vi "Do Mutate.vi"(8 "error in":errorcluster, 10 "IGene in":refnum<class "IGene.lvclass">, 11 "Binary Mutator in":refnum<class "Binary Mutator.lvclass">) -> (0 "error out":errorcluster, 2 "IGene out":refnum<class "IGene.lvclass">, 3 "Binary Mutator out":refnum<class "Binary Mutator.lvclass">)   [LabVIEW 2016, in "Binary Mutator.lvclass"]
uses:
  Binary Mutator.lvclass
  C:/Users/J51654/My Projects/Evolutionary Programming/GA Framework/GA Core/GA Core.lvclass
  IGene/IGene.lvclass
  GA Core.lvclass/GA Core.ctl
  IGene/Children/Binary/Binary Gene.lvclass
  C:/Users/J51654/My Projects/Evolutionary Programming/GA Framework/IGene/IGene.lvclass
  IGene/Children/Binary/Binary Gene.lvclass/Binary Gene.ctl
  <vilib>/Utility/error.llb/Error Cluster From Error Code.vi
  <vilib>/ErrorRing/Error Ring.xnode
  GA Core.lvclass
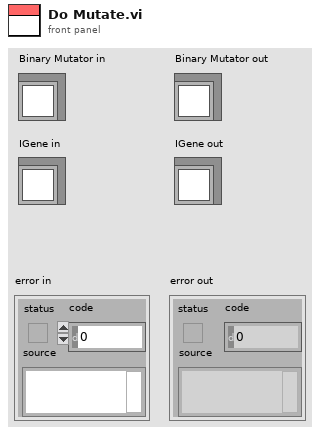
[diagram p1: front panel]
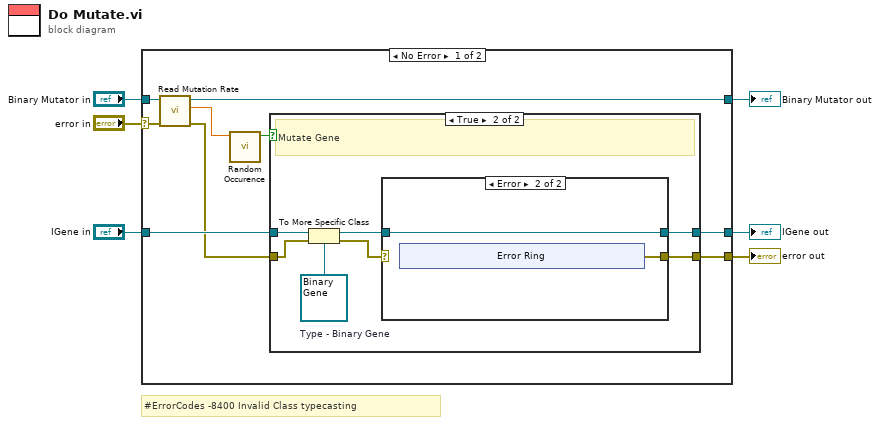
[diagram p0: block diagram]
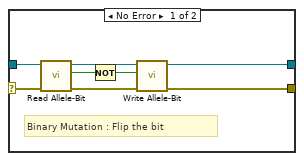
[diagram p3: hidden frame]
diagram:
  # "#ErrorCodes -8400 Invalid Class typecasting"
  n1 = case shown="No Error" "error in" {
    selector: "error in" -> [w12 w41]
    tunnel: "Binary Mutator in" -> [w15 w42]
    tunnel: "IGene in" -> [w13 w40]
    tunnel: [w14 w42] -> w3
    tunnel: [w10 w41] -> w2
    tunnel: [w9 w40] -> w1
    frame No Error {
      n2 = call "Read Mutation Rate.vi"("error in (no error)"=w12, "GA Core in"=w15) -> ("error out"=w11:errorcluster, "Mutation Rate"=w8:dbl, "GA Core out"=w14:refnum<class "Binary Mutator.lvclass">)  [unwired: 7 in]
      n3 = call "Random Occurence.vi"("Probability of Occurence (0-1)"=w8) -> ("Occured?"=w7:bool)  [unwired: 10 in]
      n4 = case shown="True" w7 {
        tunnel: w13 -> [w17 w23]
        tunnel: w11 -> [w16 w20]
        tunnel: [w16 w19] -> w10
        tunnel: [w17 w18] -> w9
        frame False {
          # "Mutation did not occur"
        }
        frame True {
          w24 = refnum<class "Binary Gene.lvclass"> refnum  # Type - Binary Gene
          # "Mutate Gene"
          n5 = To More Specific Class(target class=w24, reference=w23, error in=w20) -> (specific class reference=w22:refnum<class "Binary Gene.lvclass">, error out=w21:errorcluster)
          n6 = case shown="Error" w21 {
            selector: w21 -> [w31 _]
            tunnel: w22 -> [w32 w33]
            tunnel: [w28 w34] -> w19
            tunnel: [w29 w33] -> w18
            frame No Error {
              # "Binary Mutation : Flip the bit"
              n7 = call "Read Allele-Bit.vi"("error in (no error)"=w31, "Binary Gene in"=w32) -> ("error out"=w27:errorcluster, "Allele-Bit"=w26:bool, "Binary Gene out"=w30:refnum<class "Binary Gene.lvclass">)  [unwired: 7 in]
              n8 = Not(x=w26) -> (.not. x?=w25:bool)
              n9 = call "Write Allele-Bit.vi"("error in (no error)"=w27, "Allele-Bit"=w25, "Binary Gene in"=w30) -> ("error out"=w28:errorcluster, "Binary Gene out"=w29:refnum<class "Binary Gene.lvclass">)  [unwired: 7 in]
            }
            frame Error {
              n10 = xnode "Error Ring"() -> ("error out"=w34:errorcluster)
            }
          }
        }
      }
    }
    frame Error {
    }
  }
  "error out" <- w2
  "Binary Mutator out" <- w3
  "IGene out" <- w1
